vi "GetOSC.vi"(8 "error in":errorcluster) -> (0 "Error out":errorcluster, 1 "Channel info":T2, 2 "Oscilloscoper cluster":T1, 3 "Scope out":u32)   [LabVIEW 2018]
uses:
  LibTiePie.lvlib
  LabViewHS4/libtiepie.dll
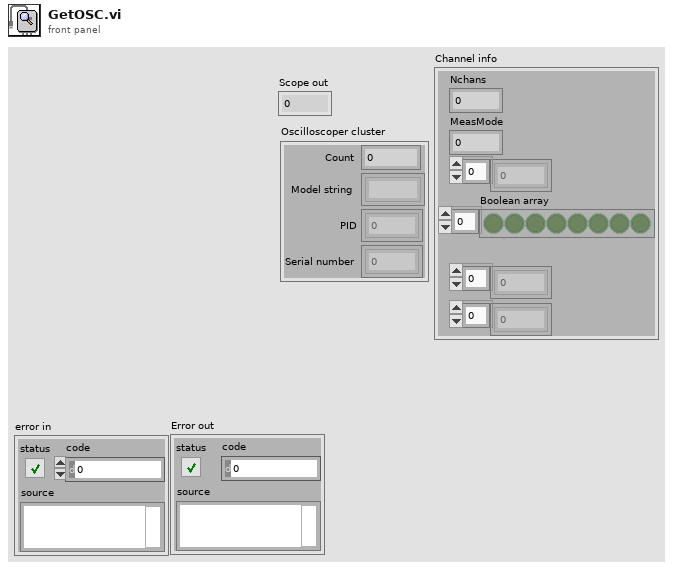
[diagram p1: front panel]
types:
  T1 = cluster{"Count":u32, "Model string":string[], "PID":u32[], "Serial number":u32[]}
  T2 = cluster{"Nchans":u16, "MeasMode":u32, dbl[], "Boolean array":bool[], u32[], dbl[]}
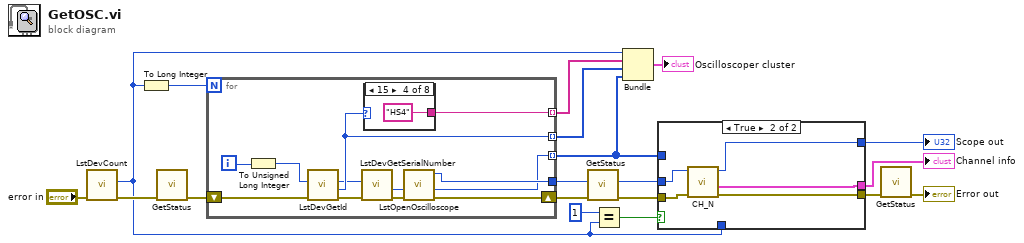
[diagram p0: block diagram]
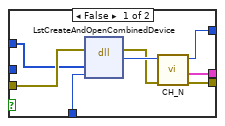
[diagram p2: hidden frame]
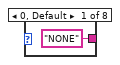
[diagram p3: hidden frame]
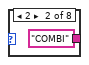
[diagram p4: hidden frame]
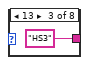
[diagram p5: hidden frame]
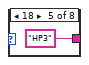
[diagram p6: hidden frame]
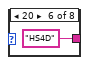
[diagram p7: hidden frame]
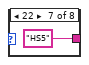
[diagram p8: hidden frame]
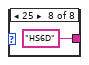
[diagram p9: hidden frame]
diagram:
  n1 = call "LstDevCount.vi"("error in (no error)"="error in") -> ("error out"=w18:errorcluster, "Count"=w6:u32)  [unwired: 9 in]
  n2 = To Long Integer(number=w6) -> (32bit integer=w17:i32)
  n3 = call "GetStatus.vi"("error in (no error)"=w18) -> ("error out"=w16:errorcluster)  [unwired: 10 in]
  n4 = for {
    N: w17 -> [_]
    tunnel: [w19] -> w2 mode=indexing
    shift-right: [w25] -> w8
    shift-left: w16 -> [w27]
    tunnel: [w24] -> w13 mode=indexing
    tunnel: [w26] -> w12 mode=indexing
    tunnel: [w20] -> w9
    i -> [w30]
    n5 = To Unsigned Long Integer(number=w30) -> (unsigned 32bit integer=w23:u32)
    n6 = call "LstDevGetId.vi"("error in (no error)"=w27, "dwId in"=w23) -> ("error out"=w28:errorcluster, "dwProductId"=w24:u32, "dwId out"=w22:u32)  [unwired: 6 in]
    n7 = call "LstDevGetSerialNumber.vi"("error in (no error)"=w28, "dwId in"=w22) -> ("error out"=w29:errorcluster, "Serial No."=w21:u32)  [unwired: 7 in, 1 out]
    n8 = case shown="15" w24 {
      tunnel: ["NONE" "COMBI" "HS3" "HS4" "HP3" "HS4D" "HS5" "HS6D"] -> w26
      frame 0, Default {
      }
      frame 2 {
      }
      frame 13 {
      }
      frame 15 {
      }
      frame 18 {
      }
      frame 20 {
      }
      frame 22 {
      }
      frame 25 {
      }
    }
    n9 = call "LstOpenOscilloscope.vi"("error in (no error)"=w29, "dwSerialNumber in"=w21) -> ("error out"=w25:errorcluster, "dwSerialNumber out"=w19:u32, "hDevice"=w20:u32)  [unwired: 7 in]
  }
  n10 = call "GetStatus.vi"("error in (no error)"=w8) -> ("error out"=w7:errorcluster)  [unwired: 10 in]
  n11 = Equal?(x=u32 1, y=w6) -> (x = y?=w11:bool)
  n12 = Bundle("Count"=w6, w12, w13, w2) -> (→"Oscilloscoper cluster":cluster{"Count":u32, string[], u32[], u32[]})  [unwired: 1 in]
  n13 = case shown="True" w11 {
    tunnel: w9 -> [_ w48]
    tunnel: w7 -> [w46 w51]
    tunnel: w2 -> [w45 _]
    tunnel: w6 -> [w44 _]
    tunnel: [w41 w50] -> w5
    tunnel: [w40 w49] -> w4
    tunnel: [w39 w47] -> w3
    frame False {
      n14 = dll-call lib="C:/Users/cwaha/Documents/LabViewHS4/libtiepie.dll" fn="LstCreateAndOpenCombinedDevice"(error in=w46, "DevH"=w45, "NDev"=w44) -> (error out=w42:errorcluster, "return type"=w43:u32)  [unwired: 4 in, 1 out]
      n15 = call "CH_N.vi"("error in (no error)"=w42, "Scope_pointer"=w43) -> ("error out"=w41:errorcluster, "Channel info"=w39:T2, "Scope out"=w40:u32)  [unwired: 5 in]
    }
    frame True {
      n16 = call "CH_N.vi"("error in (no error)"=w51, "Scope_pointer"=w48) -> ("error out"=w50:errorcluster, "Channel info"=w47:T2, "Scope out"=w49:u32)  [unwired: 5 in]
    }
  }
  "Scope out" <- w4
  "Channel info" <- w3
  n17 = call "GetStatus.vi"("error in (no error)"=w5) -> ("error out"=→"Error out":errorcluster)  [unwired: 10 in]
